vi "Update Chart.vi"(8 "error in (no error)":errorcluster, 10 "Variant":variant, 11 "MultiSubscriber in":refnum<class "MultiSubscriber.lvclass">) -> (0 "error out":errorcluster, 3 "MultiSubscriber out":refnum<class "MultiSubscriber.lvclass">)   [LabVIEW 2017, in "Integration Test Launcher.lvlib" / "TestViewables.lvlib" / "MultiSubscriber.lvclass"]
doc: "<License>\nCopyright © 2020 Tymphany, LLC | All rights reserved\nwww.Tymphany.com\nHuijun <Huijun.Guo@Tymphany.com>\n</License>"
uses:
  <vilib>/gpm_packages/@cs/example/Integration Test/MultiSubscriber/MultiSubscriber.lvclass
  C:/Program Files/National Instruments/LabVIEW 2017/vi.lib/gpm_packages/@cs/mva-viewable/Source/IViewable/IViewable/IViewable.lvclass
  <vilib>/gpm_packages/@cs/mva-viewable/Source/IViewable/IViewable/IViewable.lvclass/IViewable.ctl
  <vilib>/gpm_packages/@cs/example/Integration Test/MultiSubscriber/MultiSubscriber.lvclass/MultiSubscriber.ctl
  <vilib>/gpm_packages/@cs/mva-viewable/Source/IViewable/IViewable/IViewable.lvclass
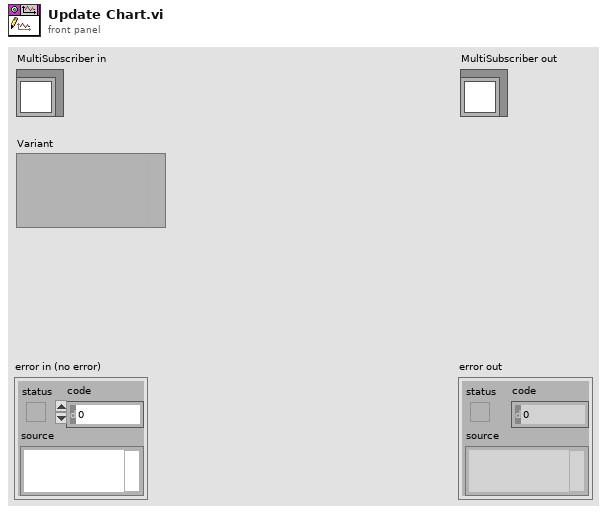
[diagram p1: front panel]
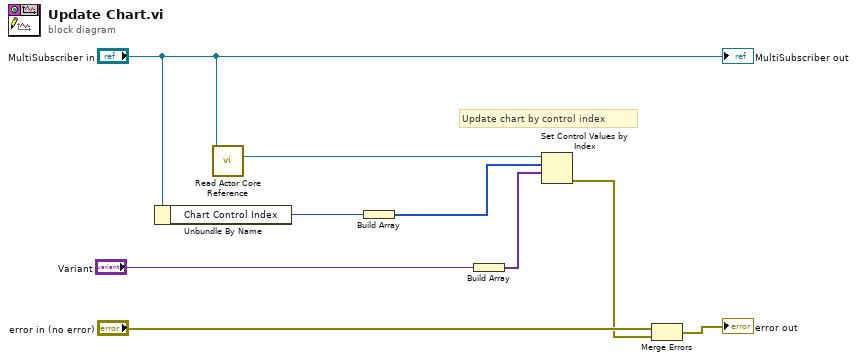
[diagram p0: block diagram]
diagram:
  # "Update chart by control index"
  n1 = Unbundle By Name("MultiSubscriber in") -> ("Chart Control Index"=w4:i32)
  n2 = call <vilib>:"Read Actor Core Reference.vi"("IViewable In"="MultiSubscriber in") -> ("Actor Core Refnum"=w7:refnum<vi>)  [unwired: 9 in, 1 out]
  n3 = Build Array(w4) -> (w3:i32[])
  n4 = Build Array("Variant") -> (w5:variant[])
  n5 = Set Control Values by Index(0:w7, 1:w3, 2:w5) -> (11:w2:errorcluster)  [unwired: 1 in]
  n6 = Merge Errors("error in (no error)", w2) -> (→"error out":errorcluster)
  "MultiSubscriber out" <- "MultiSubscriber in"
